vi "Connections Array to ConnectionList.vi"(11 "connections":T1[](array[typedef])) -> (3 "connectionList":string)   [LabVIEW 2015, in "SLSC Switch.lvlib" / "SLSC Switch.lvclass"]
uses:
  SLSC Switch.lvclass
  Controls/Connection.ctl
  slscsl/slscsl.lvclass
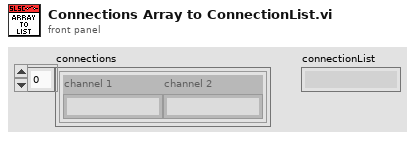
[diagram p1: front panel]
types:
  T1 = typedef "SLSC Switch.lvlib/SLSC Switch.lvclass/Connection.ctl" = cluster{"channel 1":string, "channel 2":string}
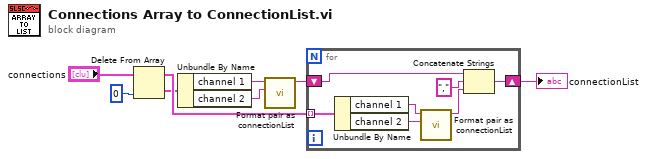
[diagram p0: block diagram]
diagram:
  n1 = Delete From Array(array="connections", index=0) -> (deleted portion=w5:T1, array with subset deleted=w6:T1[])  [unwired: 1 in]
  n2 = Unbundle By Name(w5) -> ("channel 1"=w2:string, "channel 2"=w1:string)
  n3 = call "Format pair as connectionList.vi"("channel in"=w1, "channel 1"=w2) -> ("connectionList"=w7:string)  [unwired: 9 in]
  n4 = for {
    tunnel: w6 -> [w15] mode=indexing
    shift-right: [w9] -> w8
    shift-left: w7 -> [w11]
    n5 = Unbundle By Name(w15) -> ("channel 1"=w14:string, "channel 2"=w13:string)
    n6 = call "Format pair as connectionList.vi"("channel in"=w13, "channel 1"=w14) -> ("connectionList"=w10:string)  [unwired: 9 in]
    n7 = Concatenate Strings(w11, "," ("string"), w10) -> (w9:string)
  }
  "connectionList" <- w8
